vi "Lid Lock Handling During Locked Rotor.vi"(0 "GEA2 Reference In":refnum<k24>, 11 "Error In":errorcluster) -> (4 "GEA2 Reference Out":refnum<k24>, 6 "Pass/Fail?":bool, 8 "Report Text":string, 10 "Results":dbl[][](array[numeric])=[[243.994, 0.02, 2.505, 0.02, 2.505, 0.021, 2.513, 0.021, 3.4010000000000002]], 15 "Error Out":errorcluster)   [LabVIEW 2016, in "TL27.lvlib"]
uses:
  Projects/TL27.lvlib
  C:/Automation/DLLs/PC Dot Net/GeaCommunication.dll
  Common/LabVIEW GEA2 Toolkit/LabVIEW_GEA2_Toolkit.lvlibp/type defs/Source_Destination.ctl
  Valew Common/type defs/Motor Control Without Stop Start.ctl
  <vilib>/DAQmx/read.llb/DAQmx Read (Digital Wfm 1Chan NSamp).vi
  <vilib>/DAQmx/create/channels.llb/DAQmx Create Channel (DI-Digital Input).vi
  <vilib>/DAQmx/configure/timing.llb/DAQmx Timing (Sample Clock).vi
  <vilib>/DAQmx/miscellaneous.llb/DAQmx Fill In Error Info.vi
  Common/LabVIEW GEA2 Toolkit/LabVIEW_GEA2_Toolkit.lvlibp
panel:
  in  "Low Limits":dbl[][](array[numeric])=[[230.0, 0.016, 1.0, 0.016, 1.0, 0.016, 1.0, 0.016, 0.0]]
  in  "High Limits":dbl[][](array[numeric])=[[250.0, 0.034, 3.0, 0.034, 3.0, 0.034, 3.0, 0.034, 17.5]]
  out "Digital Waveform Graph":digitalwaveform(graph)={"t0"=timestamp(3515668544.002573 s since 1904-01-01), "dt"=0.001, "Y"={"transitions"=[], "data"=array255000x1[255000 elements]}, "attributes"=variant("NI_ChannelName"=variant(string "9401_1/port0/line2"), "NI_LineNames"=variant(string "9401_1/port0/line2"))}
  in  "Standalone?":bool
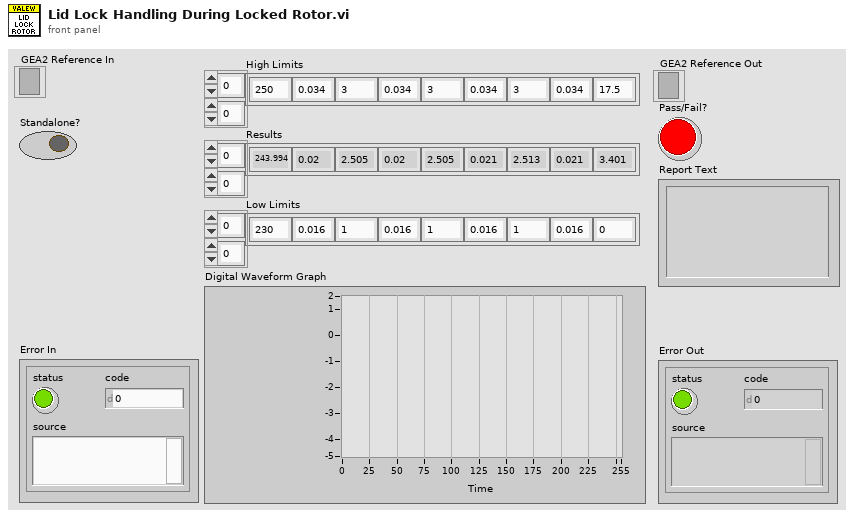
[diagram p1: front panel]
types:
  T1 = typedef "TL27.lvlib/Motor Control Without Stop Start.ctl" = cluster{"Speed (RPM)":i16, "Motor Profile Mode":u16, "Acceleration":i16, "Angle (Degrees)":i16, "Amplitude (%)\n-CCW +CW":i16}
  T2 = typedef "LabVIEW_GEA2_Toolkit.lvlibp/Source_Destination.ctl" = cluster{"Source":u8, "Destination":u8}
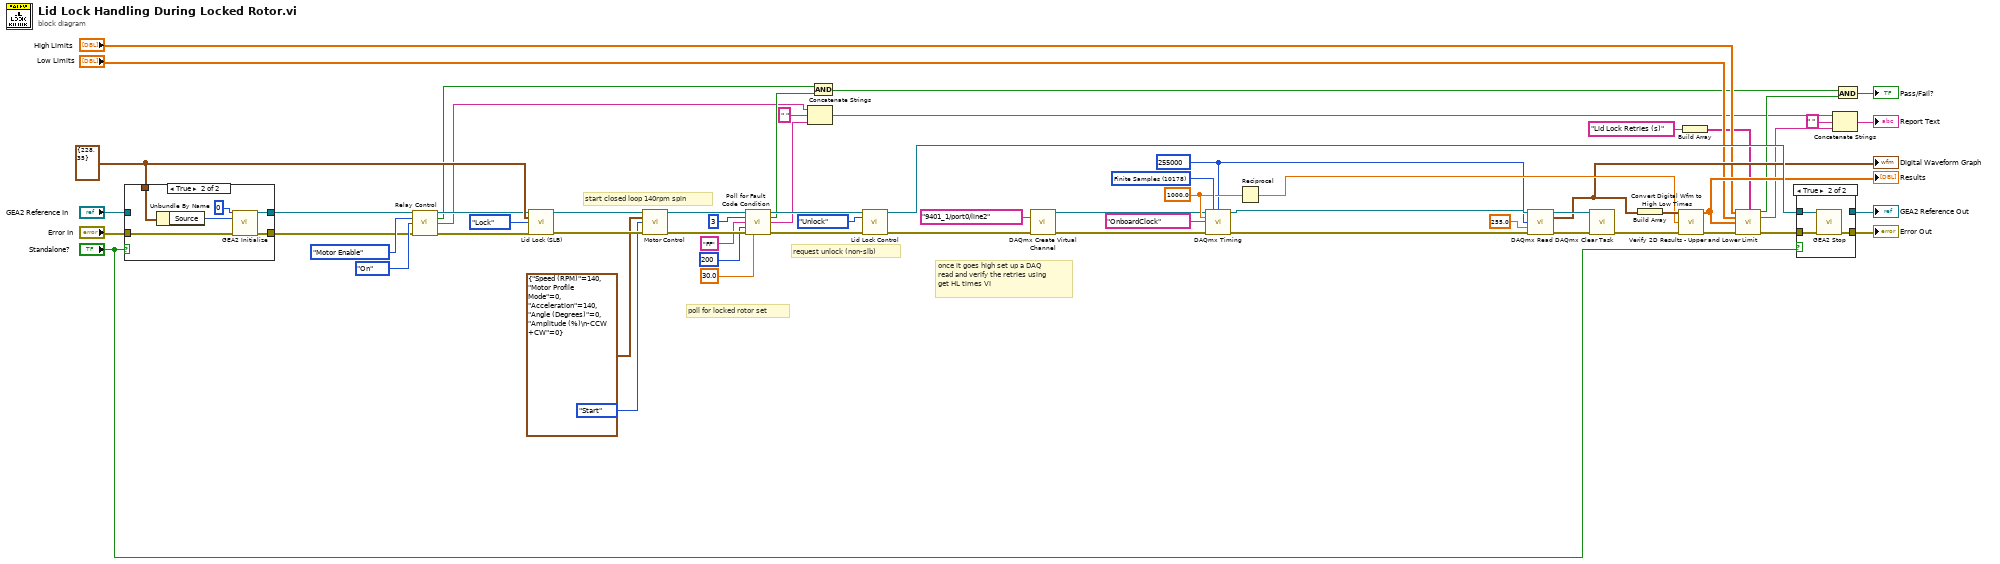
[diagram p0: block diagram]
diagram:
  w62 = 10178 items=["Finite Samples"=10178, "Continuous Samples"=10123, "Hardware Timed Single Point"=12522] ("sample mode")
  w20 = 255000 ("samples per channel")
  w59 = 1000.0 ("rate")
  w53 = T2 {"Source"=228, "Destination"=35} ("GEA Inputs")
  # "start closed loop 140rpm spin"
  # "request unlock (non-slb)"
  # "poll for locked rotor set"
  # "once it goes high set up a DAQ\nread and verify the retries using\nget HL times VI"
  n1 = case shown="True" "Standalone?" {
    tunnel: "Error In" -> [w64 w71]
    tunnel: [w64 w70] -> w32
    tunnel: "GEA2 Reference In" -> [w65 _]
    tunnel: [w65 w69] -> w54
    tunnel: w53 -> [_ w67]
    frame False {
    }
    frame True {
      n2 = Unbundle By Name(w67) -> ("Source"=w68:u8)
      n3 = call "GEA2 Initialize.vi"("Board Index"=0, "Source Address"=w68, "error in"=w71) -> ("GEA2 Reference Out"=w69:refnum<k24>, "error out"=w70:errorcluster)  [unwired: 10 in, 1 out]
    }
  }
  n4 = call "Relay Control.vi"("GEA2 Reference In"=w54, "Relay"=enum16{"Motor Enable", "Valve", "Both"}."Motor Enable", "State"=enum16{"On", "Off"}."On", "Error In"=w32) -> ("GEA2 Reference Out"=w39:refnum<k24>, "Pass/Fail?"=w3:bool, "Report Text"=w4:string, "Error Out"=w44:errorcluster)  [unwired: 8 in]
  n5 = call "Lid Lock (SLB).vi"("GEA2 Reference In"=w39, "GEA Inputs"=w53, "Action"=enum16{"Unlock", "Lock"}."Lock", "Error In"=w44) -> ("GEA2 Reference Out"=w40:refnum<k24>, "Error Out"=w50:errorcluster)  [unwired: 8 in, 2 out]
  n6 = call "Motor Control.vi"("GEA2 Reference In"=w40, "Motor Control"=T1 {"Speed (RPM)"=140, "Motor Profile Mode"=0, "Acceleration"=140, "Angle (Degrees)"=0, "Amplitude (%)\n-CCW +CW"=0}, "Action"=enum16{"Start", "Stop"}."Start", "Error In"=w50) -> ("GEA2 Reference Out"=w41:refnum<k24>, "Error Out"=w43:errorcluster)  [unwired: 10 in]
  n7 = call "Poll for Fault Code Condition.vi"("GEA2 Reference In"=w41, "Fault ID (Decimal)"=u16 3, "Fault Status (00/FF)"="FF", "Query Rate (ms)"=u32 200, "Error In"=w43, "Timeout (s)"=30.0) -> ("GEA2 Reference Out"=w34:refnum<k24>, "Pass/Fail?"=w14:bool, "Report Text"=w11:string, "Error Out"=w42:errorcluster)  [unwired: 5 in, 1 out]
  n8 = Concatenate Strings(w4, " " ("string"), w11) -> (w1:string)
  n9 = And(x=w3, y=w14) -> (x .and. y?=w2:bool)
  n10 = call "Lid Lock Control.vi"("GEA2 Reference In"=w34, "Action"=enum16{"Lock", "Unlock"}."Unlock", "Error In"=w42) -> ("GEA2 Reference Out"=w30:refnum<k24>, "Error Out"=w25:errorcluster)  [unwired: 9 in, 2 out]
  n11 = call-poly <vilib>:"DAQmx Create Virtual Channel.vi"("lines"=tag "9401_1/port0/line2", "error in"=w25) -> ("task out"=w22:refnum<k21>, "error out"=w21:errorcluster)  [unwired: 12 in]
  n12 = call-poly <vilib>:"DAQmx Timing.vi"("task/channels in"=w22, "sample mode"=w62, "samples per channel"=w20, "rate"=w59, "source"=tag "OnboardClock", "error in"=w21) -> ("task out"=w23:refnum<k21>, "error out"=w24:errorcluster)  [unwired: 8 in]
  n13 = Reciprocal(x=w59) -> (1/x=w58:dbl)
  n14 = call-poly <vilib>:"DAQmx Read.vi"("task/channels in"=w23, "number of samples per channel"=w20, "timeout"=255.0, "error in"=w24) -> ("task out"=w56:refnum<k21>, "data"=w27:digitalwaveform, "error out"=w57:errorcluster)  [unwired: 9 in]
  "Digital Waveform Graph" <- w27
  n15 = call <vilib>:"DAQmx Clear Task.vi"("task in"=w56, "error in"=w57) -> ("error out"=w55:errorcluster)  [unwired: 13 in]
  n16 = Build Array(w27) -> (w60:digitalwaveform[])
  n17 = call "Convert Digital Wfm to High Low Times.vi"("Digital Waveform In"=w60, "Dt"=w58, "Error In"=w55) -> ("HL Raw Output"=w19:dbl[][], "Error Out"=w16:errorcluster)  [unwired: 11 in]
  "Results" <- w19
  n18 = Build Array("Lid Lock Retries (s)" ("String")) -> (w12:string[])
  n19 = call "Verify 2D Results - Upper and Lower Limit.vi"("Upper Limits"="High Limits", "Array of Names"=w12, "Lower Limits"="Low Limits", "Results"=w19, "Error In"=w16) -> ("Pass/Fail?"=w7:bool, "Report Text"=w6:string, "Error Out"=w15:errorcluster)  [unwired: 7 in, 1 out]
  n20 = case shown="True" "Standalone?" {
    tunnel: w15 -> [w73 w76]
    tunnel: [w73 w75] -> w31
    tunnel: [w72 _] -> w28
    tunnel: w30 -> [w72 w74]
    frame False {
    }
    frame True {
      n21 = call "GEA2 Stop.vi"("GEA2 Reference In"=w74, "Error In"=w76) -> ("Error Out"=w75:errorcluster)  [unwired: 13 in]
    }
  }
  "GEA2 Reference Out" <- w28
  "Error Out" <- w31
  n22 = Concatenate Strings(w1, " " ("string"), w6) -> (→"Report Text":string)
  n23 = And(x=w2, y=w7) -> (x .and. y?=→"Pass/Fail?":bool)
